vi "sub_EncoderToDegrees.vi"(11 "Angle (Encoder)":dbl) -> (3 "Angle (Degrees)":dbl)   [LabVIEW 2016, in "Project 2 LabVIEW.lvrbt"]
uses:
  Project 2 LabVIEW.lvrbt
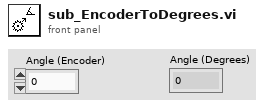
[diagram p1: front panel]
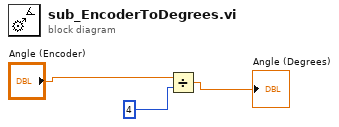
[diagram p0: block diagram]
diagram:
  n1 = Divide(x="Angle (Encoder)", y=4) -> (x/y=→"Angle (Degrees)":dbl)
